vi "Get On Off.vi"(8 "error in (no error)":errorcluster, 11 "simple Class in":refnum<class "Simple Class.lvclass">) -> (0 "error out":errorcluster, 2 "on-off":bool, 3 "simple Class out":refnum<class "Simple Class.lvclass">)   [LabVIEW 2023, in "Simple Class.lvclass"]
doc: "Get \"on-off.\""
uses:
  Simple Class.lvclass
  Simple Class.lvclass/Simple Class.ctl
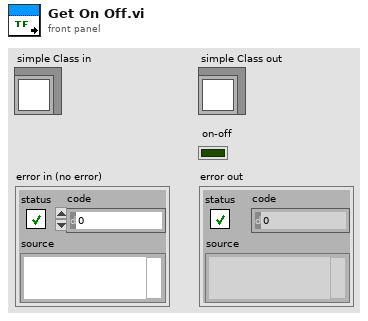
[diagram p1: front panel]
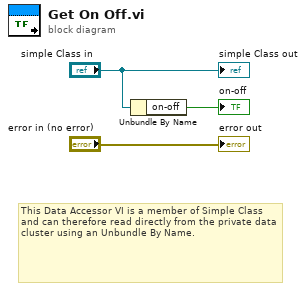
[diagram p0: block diagram]
diagram:
  # "This Data Accessor VI is a member of Simple Class and can therefore read directly from the private data cluster using an Unbundle By Name."
  n1 = Unbundle By Name("simple Class in") -> ("on-off"=→"on-off":bool)
  "simple Class out" <- "simple Class in"
  "error out" <- "error in (no error)"
